vi "GetPowerMeasurement.vi"(7 "Frequency (Hz)":dbl=100000000.0 format="%#_6p", 8 "error in (no error)":errorcluster, 9 "Level (dBm)":dbl format="%#_13g", 10 "Alias":string="PwrSensor_1", 11 "Instrument in":refnum<class "Instrument.lvclass">) -> (0 "error out":errorcluster, 2 "Power (dBm)":dbl, 3 "Instrument out":refnum<class "Instrument.lvclass">)   [LabVIEW 2014, in "Instrument.lvclass"]
uses:
  Instrument.lvclass
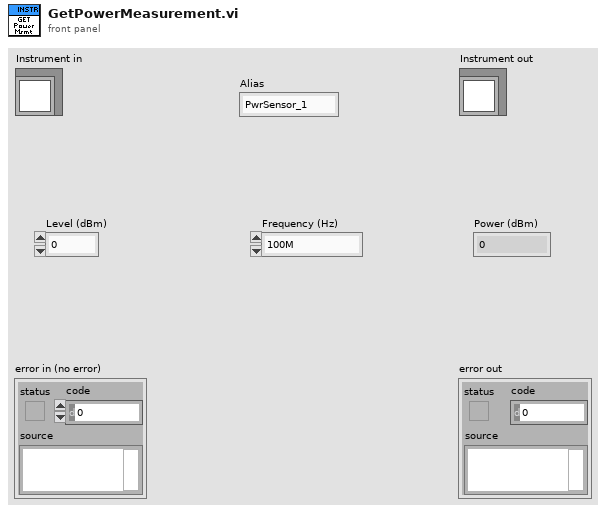
[diagram p1: front panel]
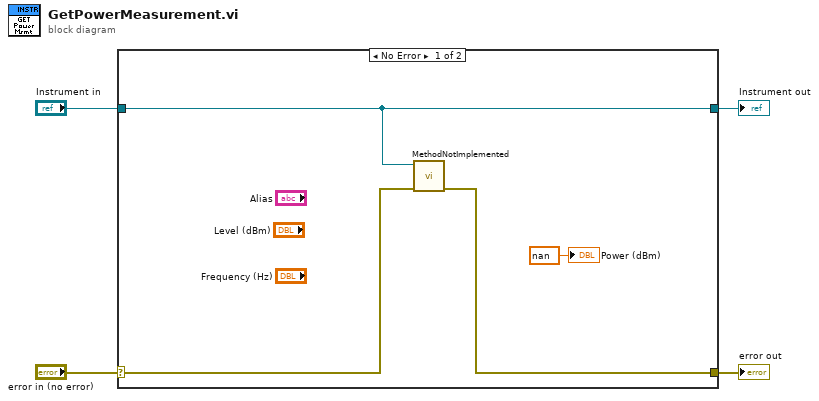
[diagram p0: block diagram]
diagram:
  n1 = case shown="No Error" "error in (no error)" {
    selector: "error in (no error)" -> [w7 w10]
    tunnel: [w6 w10] -> w3
    tunnel: [w8 w9] -> w1
    tunnel: "Instrument in" -> [w8 w9]
    frame No Error {
      n2 = call "MethodNotImplemented.vi"("error in (no error)"=w7, "LabVIEW Object In"=w8) -> ("error out"=w6:errorcluster)  [unwired: 9 in]
      "Power (dBm)" <- nan ("Power (dBm)")
    }
    frame Error {
    }
  }
  "error out" <- w3
  "Instrument out" <- w1
